vi "Read Data.vi"(0 "(FPSZ)":refnum<class "(FPSZ).lvclass">) -> (2 "Border Spacing Out":i16, 4 "Position Out":T2, 5 "Bounds Out":T1)   [LabVIEW 2016, in "(FPSZ).lvclass"]
uses:
  (FPSZ).lvclass
  <vilib>/Utility/miscctls.llb/LVPositionTypeDef.ctl
  <vilib>/Utility/miscctls.llb/LVBoundsTypeDef.ctl
  (FPSZ).lvclass/(FPSZ).ctl
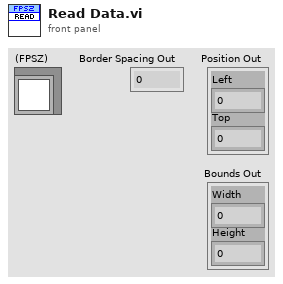
[diagram p1: front panel]
types:
  T1 = typedef "LVBoundsTypeDef.ctl" = cluster{"Width":u32, "Height":u32}
  T2 = typedef "LVPositionTypeDef.ctl" = cluster{"Left":i32, "Top":i32}
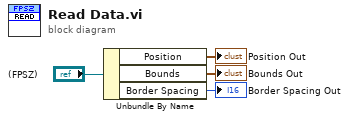
[diagram p0: block diagram]
diagram:
  n1 = Unbundle By Name("(FPSZ)") -> ("Position"=→"Position Out":T2, "Bounds"=→"Bounds Out":T1, "Border Spacing"=→"Border Spacing Out":i16)
